vi "StartIf.vi"(9 "Comparison":string(combo)="True", 11 "Data In":T1) -> (0 "False Out":T1={"Port"="", "All Code"="Hi"}, 3 "True Out":T1={"Port"="", "All Code"="Hi"})   [LabVIEW 2016]
uses:
  uPythonX/PythonData.ctl
  uPythonX/uPythonX.xctl
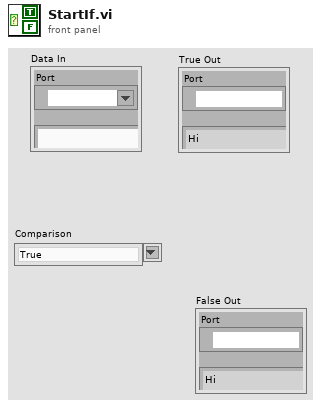
[diagram p1: front panel]
types:
  T1 = typedef "uPythonX.xctl/PythonData.ctl" = cluster{"Port":refnum<visa-resource-name>, "All Code":string}
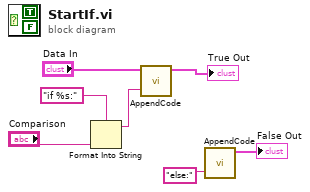
[diagram p0: block diagram]
diagram:
  n1 = Format Into String(format string="if %s:", "Comparison") -> (resulting string=w3:string)  [unwired: 2 in, 1 out]
  n2 = call "AppendCode.vi"("New Code"=w3, "Data In"="Data In") -> ("Data Out"=→"True Out":T1)  [unwired: 9 in]
  n3 = call "AppendCode.vi"("New Code"="else:" ("format string")) -> ("Data Out"=→"False Out":T1)  [unwired: 10 in]
